vi "Read filter.vi"(8 "error in (no error)":errorcluster, 11 "CRDS in":refnum<class "CRDS.lvclass">) -> (0 "error out":errorcluster, 2 "Switch.lvclass":refnum<class "Switch.lvclass">, 3 "CRDS out":refnum<class "CRDS.lvclass">)   [LabVIEW 2013, in "CRDS.lvclass"]
uses:
  CRDS.lvclass
  Switch/Switch.lvclass
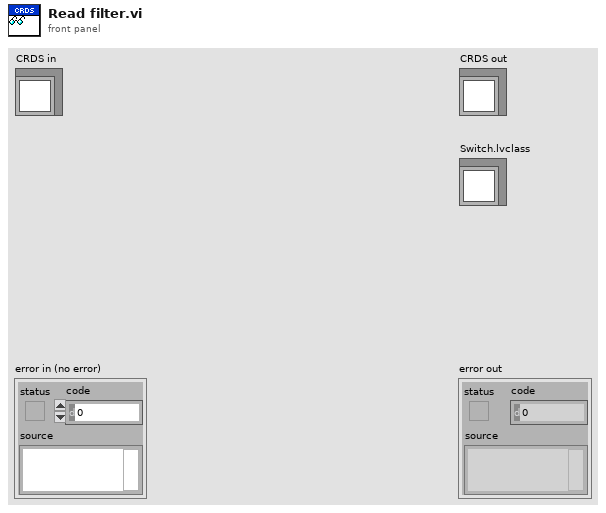
[diagram p1: front panel]
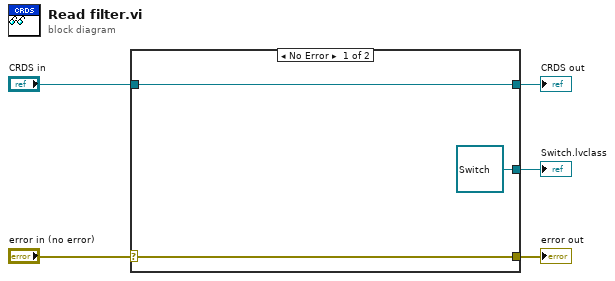
[diagram p0: block diagram]
diagram:
  n1 = case shown="No Error" "error in (no error)" {
    selector: "error in (no error)" -> [w8 w9]
    tunnel: [w8 w9] -> w4
    tunnel: [w7 w10] -> w2
    tunnel: "CRDS in" -> [w7 w10]
    tunnel: [refnum<class "Switch.lvclass"> refnum ("filter") _] -> w1
    frame No Error {
    }
    frame Error {
    }
  }
  "error out" <- w4
  "CRDS out" <- w2
  "Switch.lvclass" <- w1
